vi "createEdge_labview.vi"(9 "node 2":dbl[](array[numeric]), 10 "node1":dbl[](array[numeric]), 11 "Map":T1) -> (2 "Distance No COMPLEX":dbl, 3 "FreePath":bool)   [LabVIEW 2009]
uses:
  <vilib>/Analysis/Matrix/Datatypes/RealMatrix.ctl
  <vilib>/Analysis/Matrix/NI_Matrix.lvlib
panel:
  out "Numeric":i32
  out "COMPLEX":dbl
  out "Distance":dbl
  out "negY":dbl
  out "negX":dbl
  out "maxDist":dbl
  out "distVertical":dbl
  out "distHorizontal":dbl
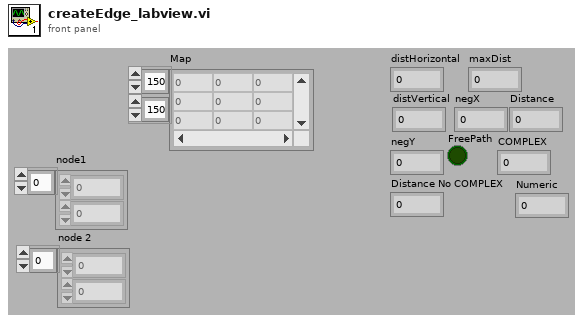
[diagram p1: front panel]
types:
  T1 = typedef "NI_Matrix.lvlib/RealMatrix.ctl" = dbl[][]
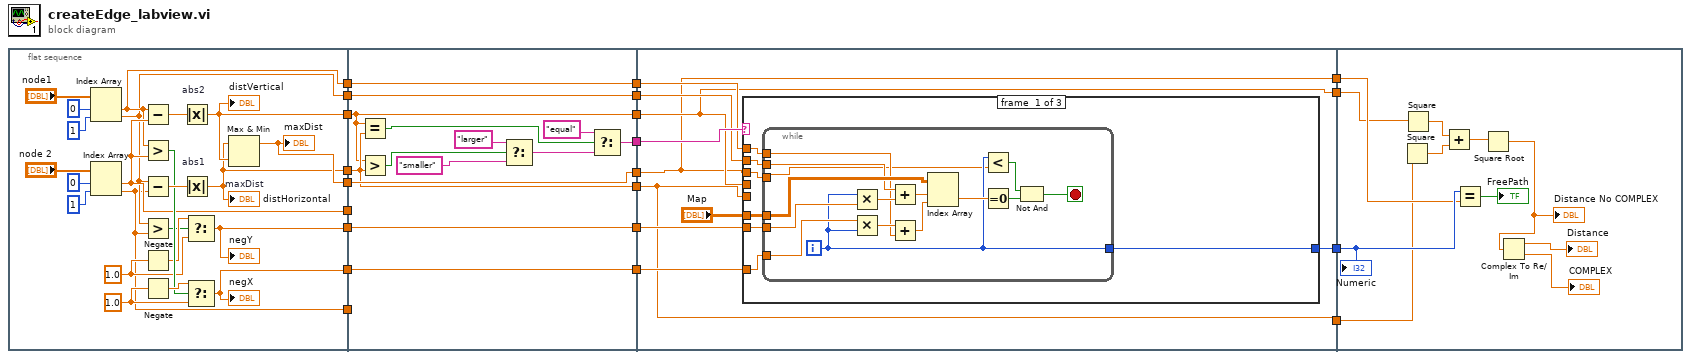
[diagram p0: block diagram]
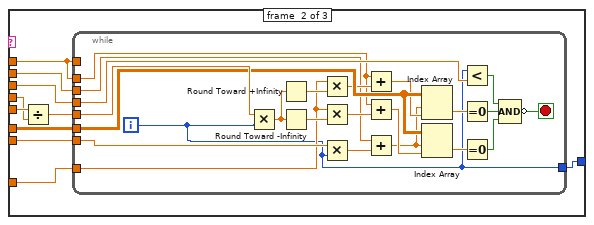
[diagram p2: hidden frame]
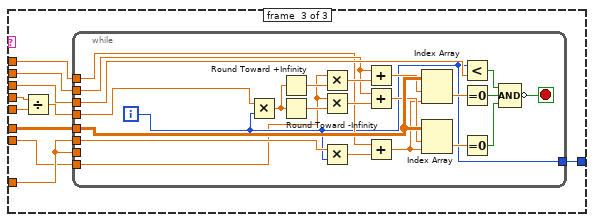
[diagram p3: hidden frame]
diagram:
  n1 = flat-sequence {
    tunnel: [w30] -> w21
    tunnel: [w29] -> w20
    tunnel: [w22] -> w19
    tunnel: [w28] -> w18
    tunnel: [w27] -> w17
    tunnel: [w26] -> w13
    tunnel: [w25] -> w12
    tunnel: [w24] -> w11
    tunnel: [w23] -> w10
    tunnel: w21 -> [w51]
    tunnel: w20 -> [w49]
    tunnel: w19 -> [w46]
    tunnel: w18 -> [w45]
    tunnel: w17 -> [w50]
    tunnel: [w55] -> w16
    tunnel: [w51] -> w15
    tunnel: [w50] -> w14
    tunnel: w13 -> [_]
    tunnel: w12 -> [w47]
    tunnel: w11 -> [w48]
    tunnel: w10 -> [_]
    tunnel: [w49] -> w9
    tunnel: [w48] -> w8
    tunnel: [w47] -> w7
    tunnel: [w46] -> w6
    tunnel: [w45] -> w5
    tunnel: w16 -> [w68]
    tunnel: w15 -> [w67]
    tunnel: w14 -> [w66]
    tunnel: w9 -> [w60]
    tunnel: w8 -> [w65]
    tunnel: w7 -> [w64]
    tunnel: w6 -> [w62]
    tunnel: w5 -> [w61]
    tunnel: [w63] -> w4
    tunnel: [w60] -> w3
    tunnel: [w62] -> w2
    tunnel: [w61] -> w1
    tunnel: w4 -> [w167]
    tunnel: w3 -> [w166]
    tunnel: w2 -> [w163]
    tunnel: w1 -> [w164]
    frame #0 {
      w31 = 1.0 ("x")
      w34 = 1.0 ("x")
      n2 = Index Array(array="node1", index #1=0 ("index"), index #2=1 ("index")) -> (element #1=w25:dbl, element #2=w24:dbl)
      n3 = Index Array(array="node 2", index #1=0 ("index"), index #2=1 ("index")) -> (element #1=w26:dbl, element #2=w23:dbl)
      n4 = Subtract(x=w25, y=w26) -> (x-y=w37:dbl)
      n5 = Greater?(x=w25, y=w26) -> (0:w35:bool)
      n6 = Subtract(x=w24, y=w23) -> (x-y=w38:dbl)
      n7 = Greater?(x=w24, y=w23) -> (0:w32:bool)
      n8 = Negate(x=w31) -> (-x=w33:dbl)
      n9 = Negate(x=w34) -> (-x=w36:dbl)
      n10 = Absolute Value "abs2"(x=w37) -> (abs(x)=w28:dbl)
      "distVertical" <- w28
      n11 = Absolute Value "abs1"(x=w38) -> (abs(x)=w22:dbl)
      "distHorizontal" <- w22
      n12 = Select(t=w33, s=w32, f=w31) -> (s? t:f=w30:dbl)
      "negY" <- w30
      n13 = Select(t=w36, s=w35, f=w34) -> (s? t:f=w27:dbl)
      "negX" <- w27
      n14 = Max & Min "maxDist"(x=w22, y=w28) -> (max(x,y)=w29:dbl)  [unwired: 1 out]
      "maxDist" <- w29
    }
    frame #1 {
      n15 = Equal?(x=w45, y=w46) -> (x = y?=w57:bool)
      n16 = Greater?(x=w45, y=w46) -> (0:w58:bool)
      n17 = Select(t="larger", s=w58, f="smaller" ("t")) -> (s? t:f=w52:string)
      n18 = Select(t="equal", s=w57, f=w52) -> (s? t:f=w55:string)
    }
    frame #2 {
      n19 = case shown="\"smaller\"" w68 {
        tunnel: "Map" -> [w75 w96 w131]
        tunnel: w67 -> [w74 w95 w124]
        tunnel: w66 -> [w73 w94 w126]
        tunnel: w60 -> [w70 w98 w133]
        tunnel: w65 -> [w72 w92 w127]
        tunnel: w64 -> [w71 w93 w125]
        tunnel: w62 -> [_ w100 w130]
        tunnel: w61 -> [_ w99 w129]
        tunnel: [w69 w91 w128] -> w63
        frame #0 {
          n20 = while {
            tunnel: w75 -> [w90]
            tunnel: w74 -> [w89]
            tunnel: w73 -> [w85]
            tunnel: w70 -> [w76]
            tunnel: w72 -> [w87]
            tunnel: w71 -> [w84]
            tunnel: [w77] -> w69
            i -> [w77]
            stop <- w80 stop-if-true
            n21 = Multiply(x=w77, y=w89) -> (x*y=w88:dbl)
            n22 = Multiply(x=w85, y=w77) -> (x*y=w86:dbl)
            n23 = Add(x=w87, y=w88) -> (x+y=w83:dbl)
            n24 = Add(x=w86, y=w84) -> (x+y=w82:dbl)
            n25 = Index Array(array=w90, index (row)=w83, index (col)=w82) -> (element=w81:dbl)
            n26 = Less?(x=w77, y=w76) -> (x < y?=w78:bool)
            n27 = Equal To 0?(x=w81) -> (x = 0?=w79:bool)
            n28 = Not And(1:w79, 2:w78) -> (0:w80:bool)
          }
        }
        frame #1 {
          n29 = Divide(x=w100, y=w99) -> (x/y=w97:dbl)
          n30 = while {
            tunnel: w98 -> [w123]
            tunnel: w97 -> [w122]
            tunnel: w96 -> [w118]
            tunnel: w95 -> [w117]
            tunnel: w94 -> [w114]
            tunnel: w93 -> [w111]
            tunnel: w93 -> [_]
            tunnel: w92 -> [w108]
            tunnel: [w101] -> w91
            i -> [w101]
            stop <- w102 stop-if-true
            n31 = Multiply(x=w122, y=w101) -> (x*y=w121:dbl)
            n32 = Round Toward +Infinity(x=w121) -> (ceil(x): smallest int >= x=w116:dbl)
            n33 = Round Toward -Infinity(1:w121) -> (0:w115:dbl)
            n34 = Multiply(x=w114, y=w116) -> (x*y=w113:dbl)
            n35 = Multiply(x=w114, y=w115) -> (x*y=w112:dbl)
            n36 = Multiply(x=w117, y=w101) -> (x*y=w120:dbl)
            n37 = Add(x=w111, y=w113) -> (x+y=w109:dbl)
            n38 = Add(x=w111, y=w112) -> (x+y=w110:dbl)
            n39 = Add(x=w108, y=w120) -> (x+y=w107:dbl)
            n40 = Index Array(array=w118, index (row)=w107, index (col)=w109) -> (element=w106:dbl)
            n41 = Index Array(array=w118, index (row)=w107, index (col)=w110) -> (element=w119:dbl)
            n42 = Less?(x=w101, y=w123) -> (x < y?=w105:bool)
            n43 = Equal To 0?(x=w106) -> (x = 0?=w104:bool)
            n44 = Equal To 0?(x=w119) -> (x = 0?=w103:bool)
            n45 = Compound Arithmetic op=AND(w105, w104, w103) -> (invert w102:bool)
          }
        }
        frame #2 {
          n46 = Divide(x=w129, y=w130) -> (x/y=w132:dbl)
          n47 = while {
            tunnel: w133 -> [w156]
            tunnel: w132 -> [w155]
            tunnel: w131 -> [w151]
            tunnel: w126 -> [w139]
            tunnel: w126 -> [_]
            tunnel: w127 -> [w146]
            tunnel: w125 -> [w145]
            tunnel: [w135] -> w128
            tunnel: w124 -> [w134]
            i -> [w135]
            stop <- w140 stop-if-true
            n48 = Multiply(x=w155, y=w135) -> (x*y=w154:dbl)
            n49 = Round Toward +Infinity(x=w154) -> (ceil(x): smallest int >= x=w150:dbl)
            n50 = Round Toward -Infinity(1:w154) -> (0:w149:dbl)
            n51 = Multiply(x=w134, y=w150) -> (x*y=w148:dbl)
            n52 = Multiply(x=w134, y=w149) -> (x*y=w147:dbl)
            n53 = Multiply(x=w139, y=w135) -> (x*y=w153:dbl)
            n54 = Add(x=w146, y=w148) -> (x+y=w138:dbl)
            n55 = Add(x=w146, y=w147) -> (x+y=w137:dbl)
            n56 = Add(x=w145, y=w153) -> (x+y=w136:dbl)
            n57 = Index Array(array=w151, index (row)=w138, index (col)=w136) -> (element=w144:dbl)
            n58 = Index Array(array=w151, index (row)=w137, index (col)=w136) -> (element=w152:dbl)
            n59 = Less?(x=w135, y=w156) -> (x < y?=w143:bool)
            n60 = Equal To 0?(x=w144) -> (x = 0?=w142:bool)
            n61 = Equal To 0?(x=w152) -> (x = 0?=w141:bool)
            n62 = Compound Arithmetic op=AND(w143, w142, w141) -> (invert w140:bool)
          }
        }
      }
    }
    frame #3 {
      n63 = Square(x=w163) -> (x^2=w161:dbl)
      n64 = Square(x=w164) -> (x^2=w162:dbl)
      n65 = Add(x=w162, y=w161) -> (x+y=w160:dbl)
      n66 = Equal?(x=w167, y=w166) -> (x = y?=→"FreePath":bool)
      n67 = Square Root(x=w160) -> (sqrt(x)=w159:dbl)
      "Distance No COMPLEX" <- w159
      n68 = Complex To Re/Im(x + iy=w159) -> (x=→"Distance":dbl, y=→"COMPLEX":dbl)
      "Numeric" <- w167
    }
  }
